vi "Get configuration chain.vi"(8 "error in (no error)":errorcluster, 11 "MeritFactorBase in":refnum<class "MeritFactor.lvclass">) -> (0 "error out":errorcluster, 1 "class name":string[](array[string]), 2 "configuration chain":variant[](array[variant]), 3 "MeritFactorBase out":refnum<class "MeritFactor.lvclass">)   [LabVIEW 2012, in "MeritFactor.lvclass"]
doc: "Returns an array of variants containing the configuration clusters of each class in the inheritance chain (lowest child class first), together with an array of all class names in the inheritance chain.\n\nFor classes without configuration cluster, the configuration chain contains empty variants."
uses:
  MeritFactor.lvclass
  <vilib>/Distrio/Murmex/Murmex/Murmex.lvclass
  MeritFactor.lvclass/MeritFactor.ctl
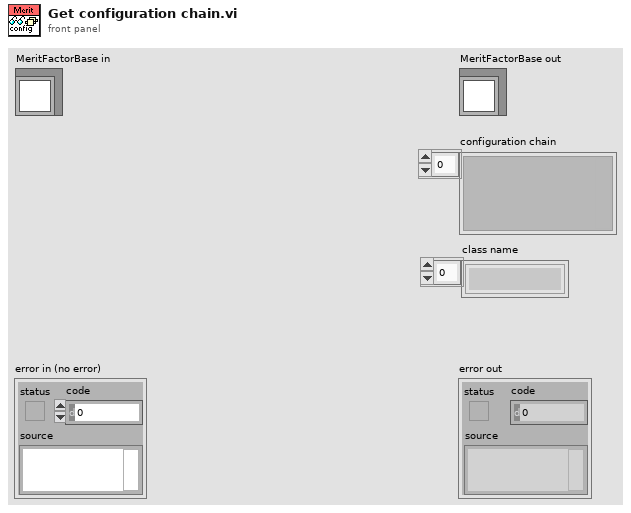
[diagram p1: front panel]
types:
  T1 = typedef "MeritFactor.lvclass/configuration cluster.ctl" = cluster{"Merit factor type":T2}
  T2 = typedef "MeritFactor.lvclass/merit factor type.ctl" = enum16{"Full frame intensity", "Brightest pixels intensity", "Contrast"}
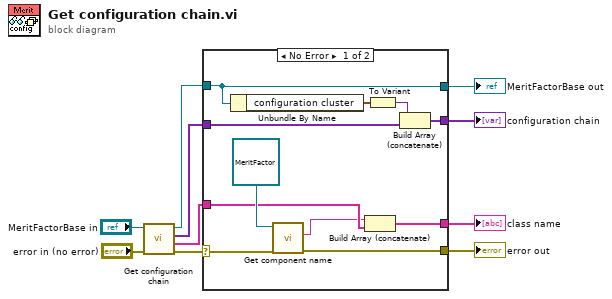
[diagram p0: block diagram]
diagram:
  n1 = call-parent "Get configuration chain.vi"("error in (no error)"="error in (no error)", "MurmexBase in"="MeritFactorBase in") -> ("error out"=w8:errorcluster, "class name"=w3:string[], "configuration chain"=w5:variant[], "MurmexBase out"=w7:refnum<class "MeritFactor.lvclass">)  [unwired: 6 in]
  n2 = case shown="No Error" w8 {
    selector: w8 -> [w21 w22]
    tunnel: w7 -> [w19 w25]
    tunnel: [w19 w25] -> w6
    tunnel: w5 -> [w17 w24]
    tunnel: [w15 w24] -> w4
    tunnel: w3 -> [w14 w23]
    tunnel: [w12 w22] -> w2
    tunnel: [w11 w23] -> w1
    frame No Error {
      n3 = Unbundle By Name(w19) -> ("configuration cluster"=w16:T1)
      n4 = call <vilib>:"Get component name.vi"("error in (no error)"=w21, "Murmex in"=refnum<class "MeritFactor.lvclass"> refnum ("MeritFactor")) -> ("error out"=w12:errorcluster, "component name"=w13:string)  [unwired: 7 in, 1 out]
      n5 = Build Array (concatenate)(w13, w14) -> (w11:string[])
      n6 = To Variant(anything=w16) -> (Variant=w18:variant)
      n7 = Build Array (concatenate)(w18, w17) -> (w15:variant[])
    }
    frame Error {
    }
  }
  "error out" <- w2
  "MeritFactorBase out" <- w6
  "configuration chain" <- w4
  "class name" <- w1
